vi "GetImageCentre (SubVI).vi"(9 "Image in \n(refnum)":T1) -> (0 "End y-line":cluster{"x":i32, dbl}, 1 "Start y-line":cluster{"x":dbl, dbl}, 2 "End x-line":cluster{dbl, "y":i32}, 3 "Start x-line":cluster{dbl, "x":dbl}, 4 "Centre Point":cluster{"X coordinate":dbl, "Y coordinate":dbl})   [LabVIEW 2016]
uses:
  <vilib>/vision/Image Controls.llb/IMAQ Image.ctl
  <resource>/objmgr/IMAQImage.rc
panel:
  # "The purpose of this\nsubVI is to compute\nthe centre coordinates\nof a given image."
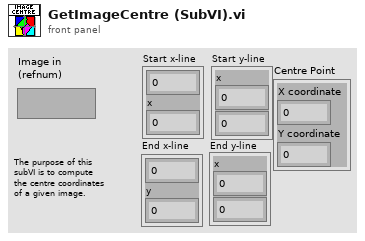
[diagram p1: front panel]
types:
  T1 = typedef "IMAQ Image.ctl" = refnum<image>
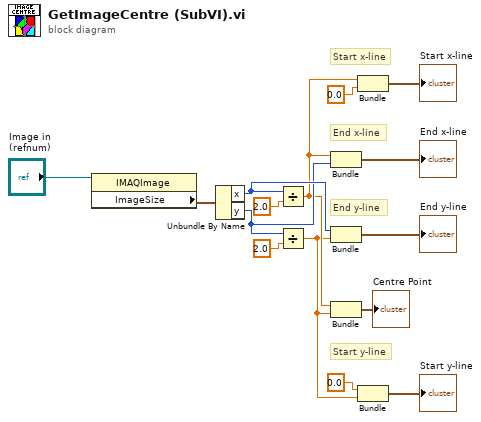
[diagram p0: block diagram]
diagram:
  # "End y-line"
  # "Start y-line"
  # "End x-line"
  # "Start x-line"
  n1 = property class="IMAQImage"(reference="Image in \n(refnum)") -> ("ImageSize"=w8:cluster{"x":i32, "y":i32})  [unwired: 1 in, 2 out]
  n2 = Unbundle By Name(w8) -> ("x"=w13:i32, "y"=w4:i32)
  n3 = Divide(x=w13, y=2.0 ("x")) -> (x/y=w2:dbl)
  n4 = Divide(x=w4, y=2.0 ("x")) -> (x/y=w1:dbl)
  n5 = Bundle(w2, "y"=w4) -> (→"End x-line":cluster{dbl, "y":i32})  [unwired: 1 in]
  n6 = Bundle("x"=w13, w1) -> (→"End y-line":cluster{"x":i32, dbl})  [unwired: 1 in]
  n7 = Bundle(w2, w1) -> (→"Centre Point":cluster{dbl, dbl})  [unwired: 1 in]
  n8 = Bundle(w2, "x"=0.0) -> (→"Start x-line":cluster{dbl, "x":dbl})  [unwired: 1 in]
  n9 = Bundle("x"=0.0, w1) -> (→"Start y-line":cluster{"x":dbl, dbl})  [unwired: 1 in]
